vi "mainPumpProbe.vi"   [LabVIEW 2017]
uses:
  globalUtilities.vi
  globalDevices.vi
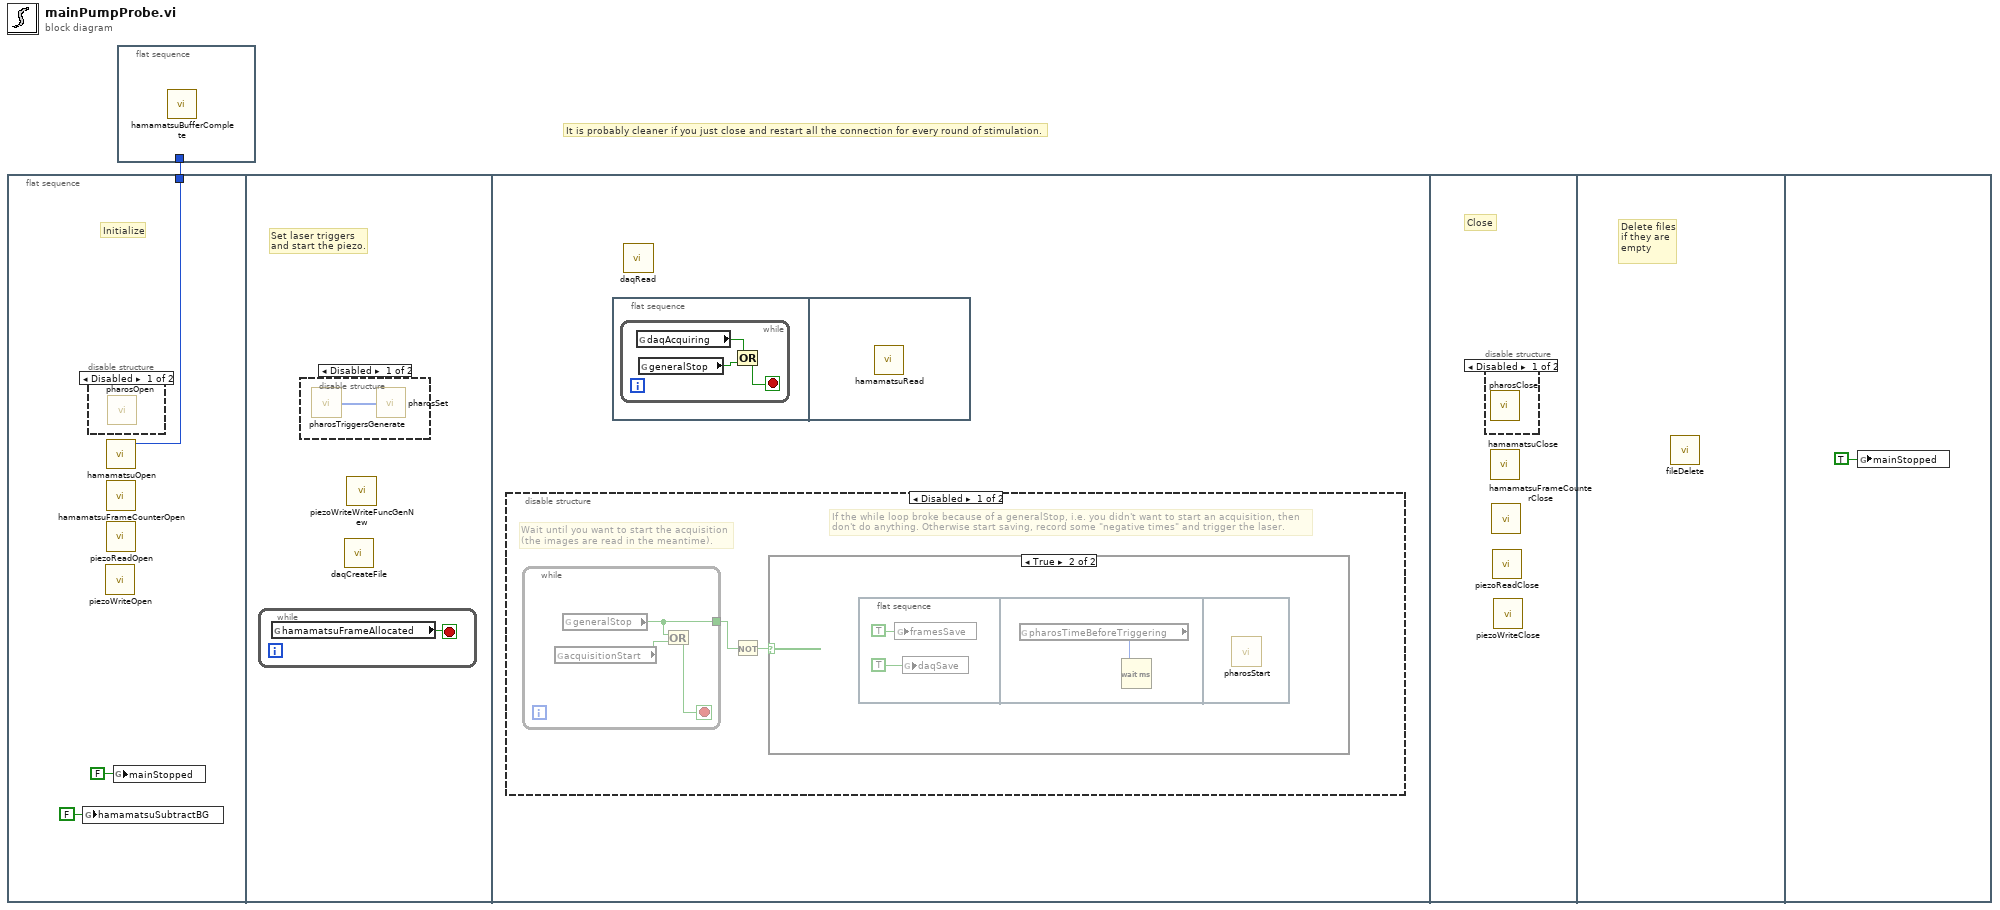
[diagram p0: block diagram]
diagram:
  # "It is probably cleaner if you just close and restart all the connection for every round of stimulation."
  n1 = flat-sequence {
    tunnel: [w2] -> w1
    frame #0 {
      # "Initialize"
      n2 = global write "globalDevices.vi" "hamamatsuSubtractBG"(FALSE ("hamamatsuSubtractBG")) -> ()
      n3 = disable-structure shown="Disabled" {
        frame Disabled {
          n4 = call "pharosOpen.vi"() -> ()  [unwired: 1 in]
        }
        frame Enabled {
        }
      }
      n5 = call "piezoWriteOpen.vi"() -> ()  [unwired: 2 in]
      n6 = call "hamamatsuOpen.vi"() -> ("Handle out"=w2:u32)  [unwired: 3 out]
      n7 = call "hamamatsuFrameCounterOpen.vi"() -> ()  [unwired: 12 in]
      n8 = call "piezoReadOpen.vi"() -> ()  [unwired: 6 in]
      n9 = global write "globalUtilities.vi" "mainStopped"(FALSE ("mainStopped")) -> ()
    }
    frame #1 {
      # "Set laser triggers\nand start the piezo."
      n10 = while {
        stop <- w5 stop-if-true
        n11 = global read "globalDevices.vi" "hamamatsuFrameAllocated"() -> (w5:bool)
      }
      n12 = disable-structure shown="Disabled" {
        frame Disabled {
          n13 = call "pharosTriggersGenerate.vi"() -> ("triggers"=w6:u8[])  [unwired: 1 in]
          n14 = call "pharosSet.vi"("triggers"=w6) -> ()
        }
        frame Enabled {
        }
      }
      n15 = call "daqCreateFile.vi"() -> ()  [unwired: 12 in]
      n16 = call "piezoWriteWriteFuncGenNew.vi"() -> ()  [unwired: 12 in]
    }
    frame #2 {
      n17 = disable-structure shown="Disabled" {
        frame Disabled {
          # "If the while loop broke because of a generalStop, i.e. you didn't want to start an acquisition, then\ndon't do anything. Otherwise start saving, record some \"negative times\" and trigger the laser."
          # "Wait until you want to start the acquisition\n(the images are read in the meantime)."
          n18 = while {
            tunnel: [w15] -> w10
            stop <- w16 stop-if-true
            n19 = global read "globalUtilities.vi" "acquisitionStart"() -> (w17:bool)
            n20 = global read "globalUtilities.vi" "generalStop"() -> (w15:bool)
            n21 = Or(x=w15, y=w17) -> (x .or. y?=w16:bool)
          }
          n22 = Not(x=w10) -> (.not. x?=w11:bool)
          n23 = case shown="True" w11 {
            frame False {
            }
            frame True {
              n24 = flat-sequence {
                frame #0 {
                  n25 = global write "globalUtilities.vi" "framesSave"(TRUE ("framesSave")) -> ()
                  n26 = global write "globalUtilities.vi" "daqSave"(TRUE ("framesSave")) -> ()
                }
                frame #1 {
                  n27 = global read "globalUtilities.vi" "pharosTimeBeforeTriggering"() -> (w14:u32)
                  n28 = Wait (ms)(milliseconds to wait=w14) -> ()  [unwired: 1 out]
                }
                frame #2 {
                  n29 = call "pharosStart.vi"() -> ()  [unwired: 12 in]
                }
              }
            }
          }
        }
        frame Enabled {
        }
      }
      n30 = flat-sequence {
        frame #0 {
          n31 = while {
            stop <- w9 stop-if-true
            n32 = global read "globalUtilities.vi" "daqAcquiring"() -> (w8:bool)
            n33 = global read "globalUtilities.vi" "generalStop"() -> (w7:bool)
            n34 = Or(x=w8, y=w7) -> (x .or. y?=w9:bool)
          }
        }
        frame #1 {
          n35 = call "hamamatsuRead.vi"() -> ()  [unwired: 12 in]
        }
      }
      n36 = call "daqRead.vi"() -> ()  [unwired: 3 in]
    }
    frame #3 {
      # "Close"
      n37 = disable-structure shown="Disabled" {
        frame Disabled {
          n38 = call "pharosClose.vi"() -> ()  [unwired: 12 in]
        }
        frame Enabled {
        }
      }
      n39 = call "hamamatsuClose.vi"() -> ()  [unwired: 1 out]
      n40 = call "hamamatsuFrameCounterClose.vi"() -> ()  [unwired: 12 in]
      n41 = call "piezoReadClose.vi"() -> ()  [unwired: 1 in]
      n42 = call "piezoWriteClose.vi"() -> ()  [unwired: 1 in]
    }
    frame #4 {
      # "Delete files\nif they are\nempty"
      n43 = call "fileDelete.vi"() -> ()  [unwired: 12 in]
    }
    frame #5 {
      n44 = global write "globalUtilities.vi" "mainStopped"(TRUE ("mainStopped")) -> ()
    }
  }
  n45 = flat-sequence {
    tunnel: w1 -> [_]
    frame #0 {
      n46 = call "hamamatsuBufferComplete.vi"() -> ()  [unwired: 12 in]
    }
  }
